vi "Status FG.vi"(8 "error in (no error)":errorcluster, 10 "Status In":string, 11 "Operation":T1) -> (0 "error out":errorcluster, 2 "Status Out":string)   [LabVIEW 2013]
uses:
  Status FG Enum.ctl
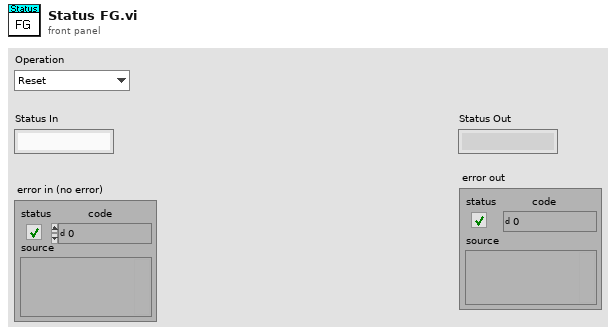
[diagram p1: front panel]
types:
  T1 = typedef "Status FG Enum.ctl" = enum16{"Reset", "Read", "Write"}
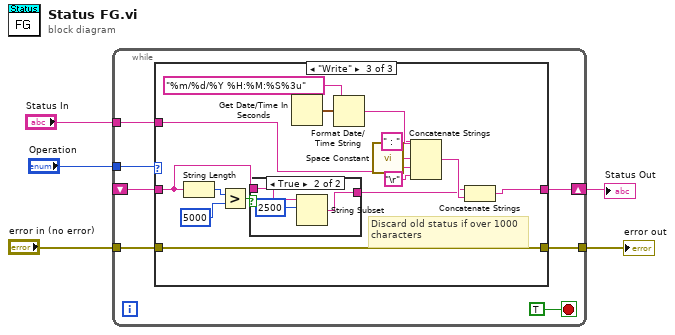
[diagram p0: block diagram]
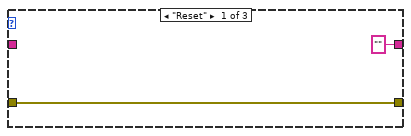
[diagram p2: hidden frame]
diagram:
  n1 = while {
    tunnel: "Operation" -> [w11]
    tunnel: "Status In" -> [w9]
    shift-right: [w10] -> w4
    shift-left: _ -> [w8]
    tunnel: [w7] -> w2
    tunnel: "error in (no error)" -> [w6]
    stop <- TRUE stop-if-true
    n2 = case shown="\"Write\"" w11 {
      tunnel: ["" ("Status In") w16 w26] -> w10
      tunnel: w9 -> [_ _ w29]
      tunnel: w8 -> [_ w16 w19]
      tunnel: [w13 w15 w25] -> w7
      tunnel: w6 -> [w13 w15 w25]
      frame "Reset" {
      }
      frame "Read" {
      }
      frame "Write" {
        # "Discard old status if over 1000\ncharacters"
        n3 = String Length(string=w19) -> (length=w22:i32)
        n4 = Greater?(x=w22, y=5000) -> (0:w20:bool)
        n5 = case shown="True" w20 {
          tunnel: w19 -> [w32 w35]
          tunnel: [w32 w34] -> w18
          frame False {
          }
          frame True {
            n6 = String Subset(string=w35, offset (0)=2500) -> (substring=w34:string)  [unwired: 1 in]
          }
        }
        n7 = Get Date/Time In Seconds() -> (seconds since 1Jan1904=w31:timestamp)
        n8 = Format Date/Time String(time format string (%c)="%m/%d/%Y %H:%M:%S%3u", seconds (now)=w31) -> (date/time string=w24:string)  [unwired: 1 in]
        n9 = call <vilib>:"Space Constant.vi"() -> ("String"=w30:string)
        n10 = Concatenate Strings(w24, " : " ("string"), w30, w29, "\r") -> (w27:string)
        n11 = Concatenate Strings(w18, w27) -> (w26:string)
      }
    }
  }
  "Status Out" <- w4
  "error out" <- w2
